vi "FirmwareProgramming2备份.vi"(8 "error in (no error)":errorcluster caption="错误输入（无错误）", 11 "SENSOR":T1) -> (0 "error out":errorcluster caption="错误输出", 2 "Message":string, 3 "Done?":bool)   [LabVIEW 2020]
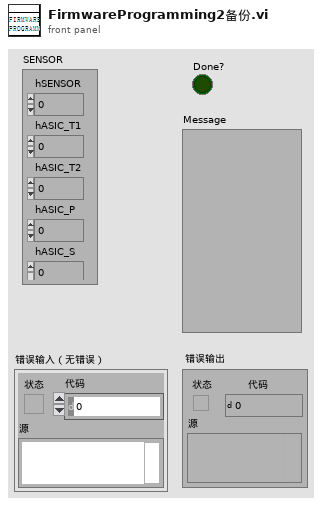
[diagram p1: front panel]
types:
  T1 = cluster{"hSENSOR":i32, "hASIC_T1":i32, "hASIC_T2":i32, "hASIC_P":i32, "hASIC_S":i32}
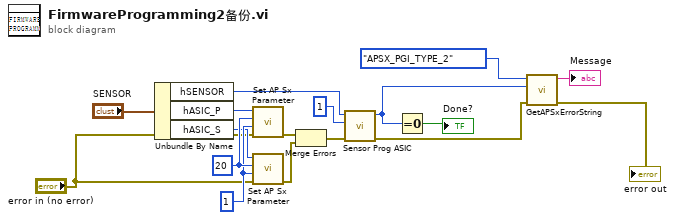
[diagram p0: block diagram]
diagram:
  w16 = 1 ("para2")
  w17 = 20 ("asicBitsName")
  n1 = Unbundle By Name("SENSOR") -> ("hSENSOR"=w11:i32, "hASIC_P"=w10:i32, "hASIC_S"=w9:i32)
  n2 = call "Set AP Sx Parameter.vi"("error in (no error)"="error in (no error)", "para2"=w16, "asicBitsName"=w17, "asicHandle"=w10) -> ("error out"=w15:errorcluster)  [unwired: 6 in, 1 out]
  n3 = call "Set AP Sx Parameter.vi"("error in (no error)"="error in (no error)", "para2"=w16, "asicBitsName"=w17, "asicHandle"=w9) -> ("error out"=w14:errorcluster)  [unwired: 6 in, 1 out]
  n4 = Merge Errors(w15, w14) -> (w12:errorcluster)
  n5 = call "Sensor Prog ASIC.vi"("error in (no error)"=w12, "progOptions"=1, "sensorHandle"=w11) -> ("error out"=w6:errorcluster, "function return"=w2:i32)  [unwired: 7 in]
  n6 = Equal To 0?(x=w2) -> (x = 0?=→"Done?":bool)
  n7 = call "GetAPSxErrorString.vi"("error in (no error)"=w6, "ErrorCode"=w2, "PGIType"=enum16{"APSX_PGI_TYPE_1", "APSX_PGI_TYPE_2"}."APSX_PGI_TYPE_2") -> ("error out"=→"error out":errorcluster, "Message"=→"Message":string)  [unwired: 7 in]
